vi "MainPIDcontrol.vi"() -> ()   [LabVIEW 2018]
uses:
  <vilib>/DAQmx/write.llb/DAQmx Write (Analog 2D DBL NChan NSamp).vi
  <vilib>/DAQmx/read.llb/DAQmx Read (Analog 2D DBL NChan NSamp).vi
  <vilib>/DAQmx/create/channels.llb/DAQmx Create Channel (AI-Voltage-Basic).vi
  <vilib>/DAQmx/create/channels.llb/DAQmx Create Channel (AO-Voltage-Basic).vi
  <vilib>/DAQmx/configure/timing.llb/DAQmx Timing (Sample Clock).vi
  <vilib>/DAQmx/miscellaneous.llb/DAQmx Fill In Error Info.vi
  <resource>/objmgr/daqmx.rc
panel:
  out "error out":errorcluster
  out "Numeric":i32
  out "NumChans":u32
  in  "SP1:":dbl(slide)=1.0 min=0.0 max=1.0 scale=-0.1..1.5
  out "MV1:":dbl(slide)=100.0 scale=-100.0..100.0
  out "PV1:":dbl(slide)=29.253567073551352 scale=0.0..1.0
  out "Actual Sample Rate":dbl=1000.0 format="%0.2f"
  in  "Stop Button":bool
  out "Process Variable and Setpoint":dbl[][](graph)
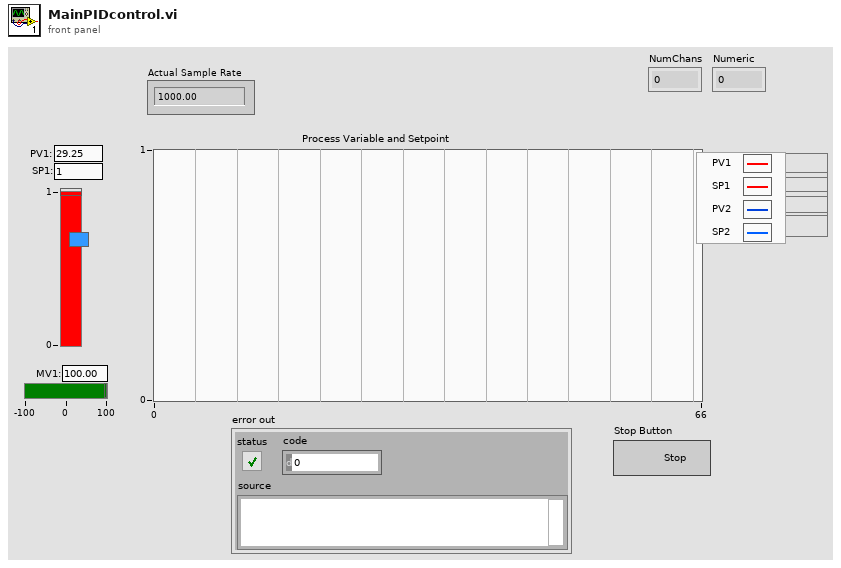
[diagram p1: front panel]
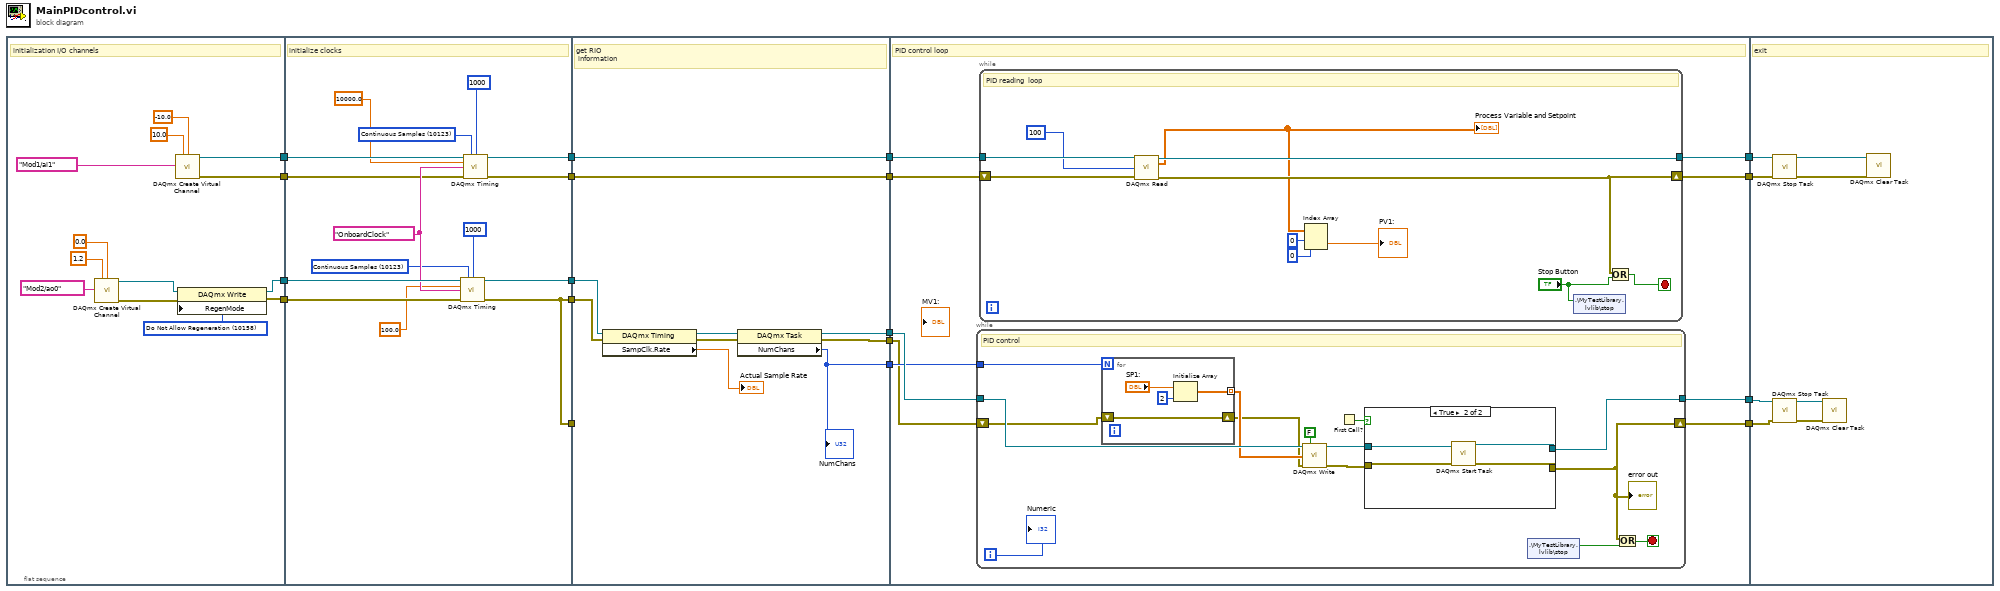
[diagram p0: block diagram]
diagram:
  n1 = flat-sequence {
    tunnel: [w29] -> w18
    tunnel: [w21] -> w17
    tunnel: [w22] -> w16
    tunnel: [w28] -> w15
    tunnel: w18 -> [w46]
    tunnel: w17 -> [w45]
    tunnel: w16 -> [w42]
    tunnel: w15 -> [w41]
    tunnel: [w36] -> w10
    tunnel: [w33] -> w9
    tunnel: [w35] -> w8
    tunnel: [w34] -> w6
    tunnel: [w33] -> w4
    tunnel: w10 -> [w51]
    tunnel: w9 -> [_]
    tunnel: w8 -> [w56]
    tunnel: [w56] -> w7
    tunnel: w6 -> [w55]
    tunnel: [w55] -> w5
    tunnel: w4 -> [w50]
    tunnel: [w49] -> w3
    tunnel: [w48] -> w2
    tunnel: [w47] -> w1
    tunnel: w7 -> [w65]
    tunnel: w5 -> [w64]
    tunnel: [w63] -> w14
    tunnel: [w62] -> w13
    tunnel: [w61] -> w12
    tunnel: [w60] -> w11
    tunnel: w3 -> [w59]
    tunnel: w2 -> [w58]
    tunnel: w1 -> [w57]
    tunnel: w14 -> [w105]
    tunnel: w13 -> [w104]
    tunnel: w12 -> [w106]
    tunnel: w11 -> [w107]
    frame #0 {
      w19 = 10158 items=["Allow Regeneration"=10097, "Do Not Allow Regeneration"=10158] ("RegenMode")
      # "initialization I/O channels"
      n2 = call-poly <vilib>:"DAQmx Create Virtual Channel.vi"("maximum value"=1.2, "minimum value"=0.0, "physical channels"=tag "Mod2/ao0") -> ("task out"=w20:refnum<k21>, "error out"=w23:errorcluster)  [unwired: 11 in]
      n3 = call-poly <vilib>:"DAQmx Create Virtual Channel.vi"("maximum value"=10.0, "minimum value"=-10.0, "physical channels"=tag "Mod1/ai1") -> ("task out"=w29:refnum<k21>, "error out"=w28:errorcluster)  [unwired: 11 in]
      n4 = property class="DAQmx Write"(reference=w20, error in=w23, "RegenMode"=w19) -> (reference out=w21:refnum<k21>, error out=w22:errorcluster)
    }
    frame #1 {
      w37 = 10123 items=["Finite Samples"=10178, "Continuous Samples"=10123, "Hardware Timed Single Point"=12522] ("sample mode")
      w38 = 10123 items=["Finite Samples"=10178, "Continuous Samples"=10123, "Hardware Timed Single Point"=12522] ("sample mode")
      w44 = tag "OnboardClock" ("source")
      # "initialize clocks"
      n5 = call-poly <vilib>:"DAQmx Timing.vi"("task/channels in"=w45, "sample mode"=w38, "samples per channel"=1000, "rate"=100.0, "source"=w44, "error in"=w42) -> ("task out"=w36:refnum<k21>, "error out"=w33:errorcluster)  [unwired: 8 in]
      n6 = call-poly <vilib>:"DAQmx Timing.vi"("task/channels in"=w46, "sample mode"=w37, "samples per channel"=1000, "rate"=10000.0, "source"=w44, "error in"=w41) -> ("task out"=w35:refnum<k21>, "error out"=w34:errorcluster)  [unwired: 8 in]
    }
    frame #2 {
      # "get RIO\n information"
      n7 = property class="DAQmx Timing"(reference=w51, error in=w50) -> (reference out=w53:refnum<k21>, error out=w52:errorcluster, "SampClk.Rate"=→"Actual Sample Rate":dbl)
      n8 = property class="DAQmx Task"(reference=w53, error in=w52) -> (reference out=w49:refnum<k21>, error out=w47:errorcluster, "NumChans"=w48:u32)
      "NumChans" <- w48
    }
    frame #3 {
      # "PID control loop"
      n9 = while {
        tunnel: w59 -> [w77]
        tunnel: [w71] -> w60
        shift-right: [w69] -> w61
        shift-left: w57 -> [w67]
        tunnel: w58 -> [w75]
        i -> [w68]
        stop <- w78 stop-if-true
        # "PID control"
        n10 = for {
          N: w75 -> [_]
          tunnel: [w88] -> w74 mode=indexing
          shift-right: [w86] -> w66
          shift-left: w67 -> [w86]
          n11 = Initialize Array("SP1:", 2 ("dimension size")) -> (w88:dbl[])
        }
        n12 = call-poly <vilib>:"DAQmx Write.vi"("task/channels in"=w77, "auto start"=FALSE, "data"=w74, "error in"=w66) -> ("task out"=w72:refnum<k21>, "error out"=w70:errorcluster)  [unwired: 9 in, 1 out]
        n13 = First Call?() -> (First Call?: T/F=w73:bool)
        n14 = case shown="True" w73 {
          tunnel: w72 -> [w81 w85]
          tunnel: [w81 w84] -> w71
          tunnel: w70 -> [w80 w83]
          tunnel: [w80 w82] -> w69
          frame False {
          }
          frame True {
            n15 = call <vilib>:"DAQmx Start Task.vi"("task/channels in"=w85, "error in"=w83) -> ("task out"=w84:refnum<k21>, "error out"=w82:errorcluster)  [unwired: 12 in]
          }
        }
        "error out" <- w69
        n16 = shared-variable ".\\MyTestLibrary.lvlib\\stop"() -> (w79:bool)  [unwired: 1 in, 1 out]
        n17 = Or(x=w69, y=w79) -> (x .or. y?=w78:bool)
        "Numeric" <- w68
      }
      n18 = while {
        tunnel: w65 -> [w98]
        tunnel: [w95] -> w63
        shift-right: [w96] -> w62
        shift-left: w64 -> [w97]
        stop <- w99 stop-if-true
        # "PID reading  loop"
        n19 = call-poly <vilib>:"DAQmx Read.vi"("task/channels in"=w98, "number of samples per channel"=100, "error in"=w97) -> ("task out"=w95:refnum<k21>, "data"=w93:dbl[][], "error out"=w96:errorcluster)  [unwired: 10 in]
        "Process Variable and Setpoint" <- w93
        n20 = Index Array(array=w93, index (row)=0, index (col)=0 ("disabled index (col)")) -> (element=→"PV1:":dbl)
        n21 = shared-variable ".\\MyTestLibrary.lvlib\\stop"("Stop Button") -> ()  [unwired: 1 in, 1 out]
        n22 = Or(x=w96, y="Stop Button") -> (x .or. y?=w99:bool)
      }
    }
    frame #4 {
      # "exit"
      n23 = call <vilib>:"DAQmx Stop Task.vi"("task/channels in"=w105, "error in"=w104) -> ("task out"=w103:refnum<k21>)  [unwired: 12 in, 1 out]
      n24 = call <vilib>:"DAQmx Stop Task.vi"("task/channels in"=w107, "error in"=w106) -> ("task out"=w102:refnum<k21>, "error out"=w101:errorcluster)  [unwired: 12 in]
      n25 = call <vilib>:"DAQmx Clear Task.vi"("task in"=w102, "error in"=w101) -> ()  [unwired: 13 in, 1 out]
      n26 = call <vilib>:"DAQmx Clear Task.vi"("task in"=w103, "error in"=w104) -> ()  [unwired: 13 in, 1 out]
    }
  }
